vi "2.10)Termometer.vi"() -> ()   [LabVIEW 2020]
panel:
  out "Термометр":dbl(slide) scale=-50.0..50.0
  in  "Выбор шкалы":i64(knob) scale=0.0..2.0
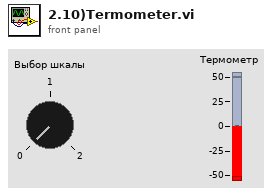
[diagram p1: front panel]
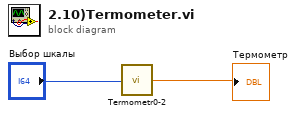
[diagram p0: block diagram]
diagram:
  n1 = call "Termometr0-2.vi"("Numeric"="Выбор шкалы") -> ("Град"=→"Термометр":dbl)
